vi "writeNexus.vi"(8 "error in (no error)":errorcluster, 10 "Command":string="I_C_1:A_C?") -> (0 "error out":errorcluster, 3 "NEXUS out":refnum<class "NEXUS.lvclass">)   [LabVIEW 2019, in "NEXUS.lvclass"]
uses:
  NEXUS.lvclass
  <vilib>/Instr/_visa.llb/VISA Configure Serial Port (Instr).vi
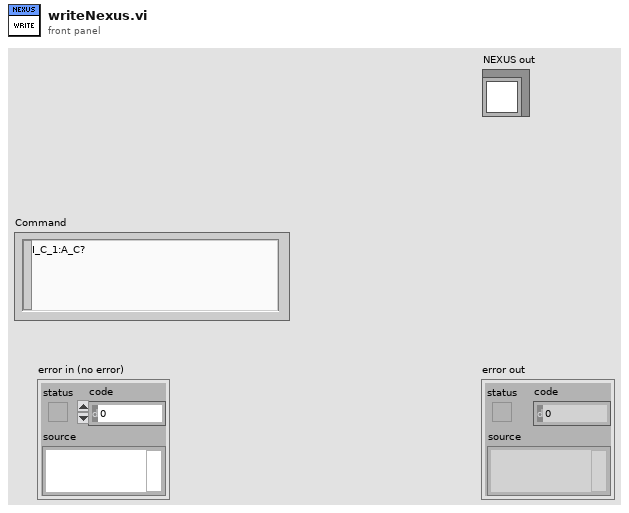
[diagram p1: front panel]
types:
  T1 = cluster{"baud rate":u32, "data bits":u16, "parity":enum16{"None", "Odd", "Even", "Mark", "Space"}, "stop bits":u16, "flow control":u16}
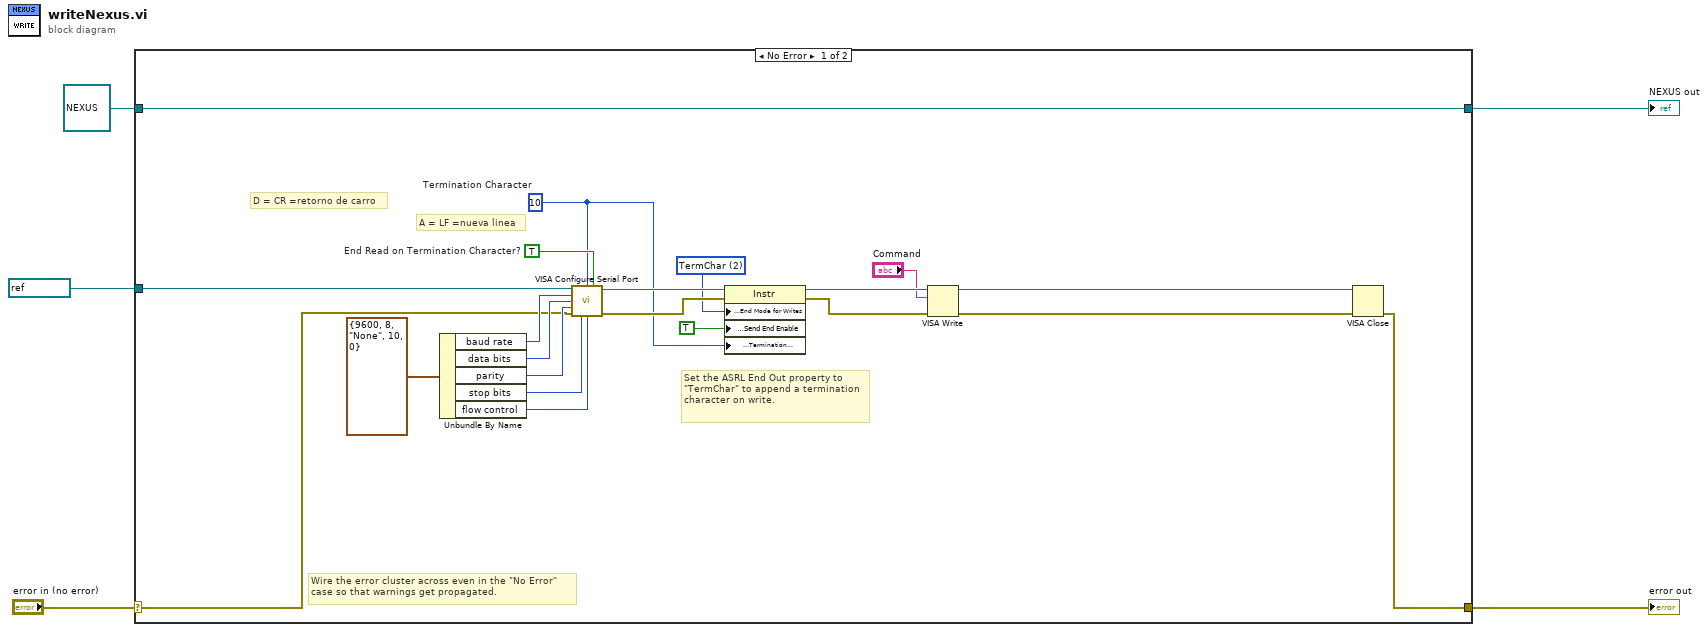
[diagram p0: block diagram]
diagram:
  n1 = case shown="No Error" "error in (no error)" {
    selector: "error in (no error)" -> [w7 w28]
    tunnel: [w6 w28] -> w4
    tunnel: [w26 w27] -> w2
    tunnel: refnum<class "NEXUS.lvclass"> refnum ("NEXUS in") -> [w26 w27]
    tunnel: refnum<visa-resource-name> "COM6" ("VISA resource name") -> [w8 _]
    frame No Error {
      w10 = u16 2 items=["None", "LastBit", "TermChar", "Break"] ("Serial Settings:Serial End Mode for Writes")
      w14 = u8 10  # Termination Character
      w18 = TRUE  # End Read on Termination Character?
      # "Set the ASRL End Out property to \"TermChar\" to append a termination character on write."
      # "D = CR =retorno de carro"
      # "A = LF =nueva linea"
      # "Wire the error cluster across even in the \"No Error\"\ncase so that warnings get propagated."
      n2 = Unbundle By Name(T1 {"baud rate"=9600, "data bits"=8, "parity"=enum."None", "stop bits"=10, "flow control"=0} ("Serial Settings")) -> ("baud rate"=w20:u32, "data bits"=w21:u16, "parity"=w22:enum16{"None", "Odd", "Even", "Mark", "Space"}, "stop bits"=w23:u16, "flow control"=w17:u16)
      n3 = call-poly "VISA Configure Serial Port"("VISA resource name"=w8, "termination char\n(0xA = '\\n' = LF)"=w14, "Enable Termination\nChar (T)"=w18, "baud rate (9600)"=w20, "data bits (8)"=w21, "parity (0:none)"=w22, "error in (no error)"=w7, "stop bits (10: 1 bit)"=w23, "flow control (0:none)"=w17) -> ("VISA resource name out"=w24:refnum<visa-resource-name>, "error out"=w25:errorcluster)  [unwired: 1 in, 4 out]
      n4 = property class="Instr"(reference=w24, error in=w25, "Serial Settings:End Mode for Writes"=w10, "Message Based Settings:Send End Enable"=TRUE, "Message Based Settings:Termination Character"=w14) -> (reference out=w15:refnum<visa-resource-name>, error out=w16:errorcluster)
      n5 = VISA Write(VISA resource name=w15, write buffer="Command", error in (no error)=w16) -> (VISA resource name out=w13:refnum<visa-resource-name>, error out=w12:errorcluster)  [unwired: 1 out]
      n6 = VISA Close(VISA resource name=w13, error in (no error)=w12) -> (error out=w6:errorcluster)
    }
    frame Error {
    }
  }
  "error out" <- w4
  "NEXUS out" <- w2
